vi "TEST-01.vi"() -> ()   [LabVIEW 2017]
panel:
  out "ปริมาตร(V)":u8
  out "พื้นที่ผิว(A)":u8
  in  "h (ฟุต)":u8
  out "h (เมตร)":dbl
  out "r (เมตร)":dbl
  in  "r (นิ้ว)":u8
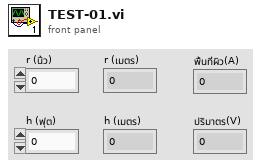
[diagram p1: front panel]
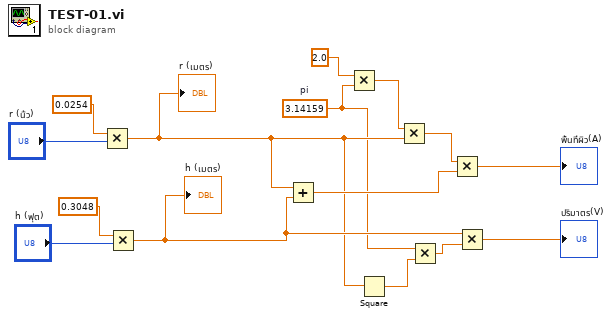
[diagram p0: block diagram]
diagram:
  w2 = 3.14159  # pi
  n1 = Multiply(x=0.0254, y="r (นิ้ว)") -> (x*y=w4:dbl)
  "r (เมตร)" <- w4
  n2 = Multiply(x=0.3048, y="h (ฟุต)") -> (x*y=w6:dbl)
  "h (เมตร)" <- w6
  n3 = Add(x=w4, y=w6) -> (x+y=w10:dbl)
  n4 = Multiply(x=2.0, y=w2) -> (x*y=w7:dbl)
  n5 = Square(x=w4) -> (x^2=w3:dbl)
  n6 = Multiply(x=w7, y=w4) -> (x*y=w9:dbl)
  n7 = Multiply(x=w2, y=w3) -> (x*y=w1:dbl)
  n8 = Multiply(x=w9, y=w10) -> (x*y=→"พื้นที่ผิว(A)":dbl)
  n9 = Multiply(x=w6, y=w1) -> (x*y=→"ปริมาตร(V)":dbl)
